vi "GraphAllData.vi"() -> ()   [LabVIEW 2014]
uses:
  <vilib>/Utility/file.llb/Read From Spreadsheet File (DBL).vi
panel:
  in  "Boolean":bool=TRUE caption="Comma - Dot"
  out "Intensity":cluster{dbl[], dbl[]}[](graph)=[{[0.4482, 0.74565, 1.03465, 1.41595, 1.6587500000000002, 2.1205, 2.3416, 2.64395, 2.8270999999999997], [2885.233184799485, 3819.39283016977, 6741.485053135704, 8371.343227868216, 10568.06564807566, 15816.573468461038, 19513.91663154004, 18468.575918850947, 21904.929929348546]}, {[0.7978500000000001, 1.1793, 1.53135, 1.9195, 2.32255, 2.59605, 2.89845, 2.9768, 3.11285], [4913.128828304257, 8837.628945556497, 14162.459131308004, 21909.101985554447, 24670.326730345823, 30736.435346877264, 29659.90767199613, 36470.26711538562, 32082.173989529885]}, {[0.75805, 1.09005, 1.47645, 1.84945, 2.21955, 2.4829000000000003, 2.7510999999999997, 2.9362, 3.0384499999999997], [2427.837864610553, 6520.525680095638, 15723.354958142441, 21679.009604909883, 27664.463875772657, 35328.219444, 30338.40494135966, 36543.11286503484, 32147.938633638245]}, {[0.8815000000000001, 1.2015500000000001, 1.51245, 1.85385, 2.2742999999999998, 2.5146499999999996, 2.71375, 2.854, 2.91995], [6950.989572736701, 14497.805584718632, 20312.386151964263, 34829.46500046118, 46881.37359550876, 60117.265315518525, 64636.230201609826, 64597.35246922127, 64607.68160946114]}]
  in  "Reduce Array Size (2^nTimes)":i32=3
  out "Filenames":string[](array[string])=["ovo-4-Spectrum Jan-07-2022 Time 03-56Analysed #1.and", "ovo-3-Spectrum Jan-07-2022 Time 03-44Analysed #1.and", "ovo-2-Spectrum Jan-07-2022 Time 03-42Analysed #1.and", "ovo-1-Spectrum Jan-07-2022 Time 03-40Analysed #1.and"]
  out "Plot Color":u32[](array[colorbox])=[483491, 16728642, 982784, 4375295]
  in  "Plot.Plot Interpolation":u8=2 max=5
  in  "Plot.Point Style":u8=2 max=16
  in  "Plot.Line Width":u8=5
  in  "Plot.Line Style":u8 max=4
  in  "Length":i32=110
  in  "Start index":i32=33
  out "FWHM":cluster{dbl[], dbl[]}[](graph)=[{[0.4482, 0.74565, 1.03465, 1.41595, 1.6587500000000002, 2.1205, 2.3416, 2.64395, 2.8270999999999997], [34.947243991883, 33.834151010707, 41.858625650798, 28.047486632265, 26.265721513935, 22.606313384127, 20.708480495843, 22.186951698272, 19.059334529408]}, {[0.7978500000000001, 1.1793, 1.53135, 1.9195, 2.32255, 2.59605, 2.89845, 2.9768, 3.11285], [33.067735928078, 24.344505399387, 19.47079873387, 12.074343500554, 15.950722154285, 12.702887849716, 16.078576237118, 9.241305141305, 15.837298026481]}, {[0.75805, 1.09005, 1.47645, 1.84945, 2.21955, 2.4829000000000003, 2.7510999999999997, 2.9362, 3.0384499999999997], [31.856003209472, 17.763577743245, 6.463072800948, 7.100905977113, 6.459600827454, 5.797900738679, 7.140966250209, 6.895364179986, 7.095295071816]}, {[0.8815000000000001, 1.2015500000000001, 1.51245, 1.85385, 2.2742999999999998, 2.5146499999999996, 2.71375, 2.854, 2.91995], [56.013195210149, 21.725458390603, 18.108405137041, 11.925527469703, 8.834451268768, 8.192653465718, 9.670319607355, 12.851225125147, 12.213374983365]}]
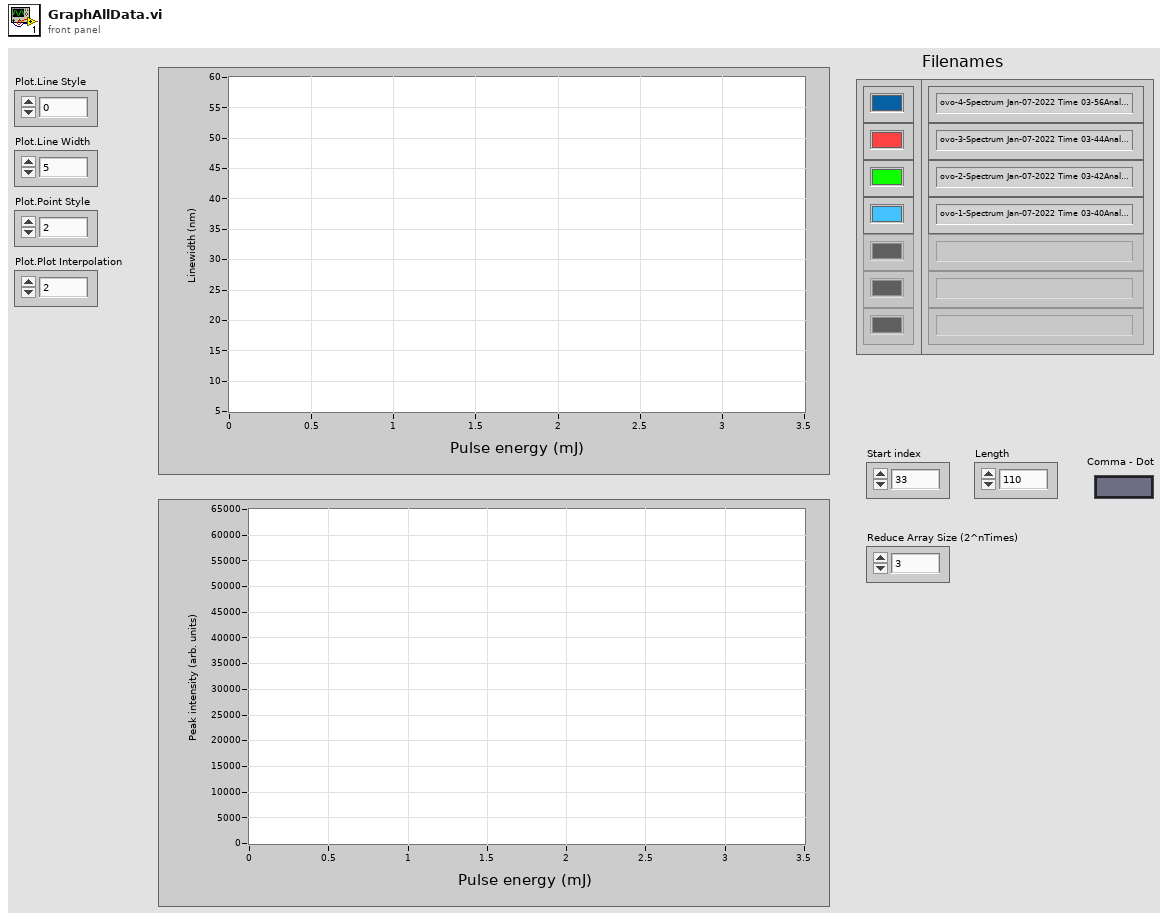
[diagram p1: front panel]
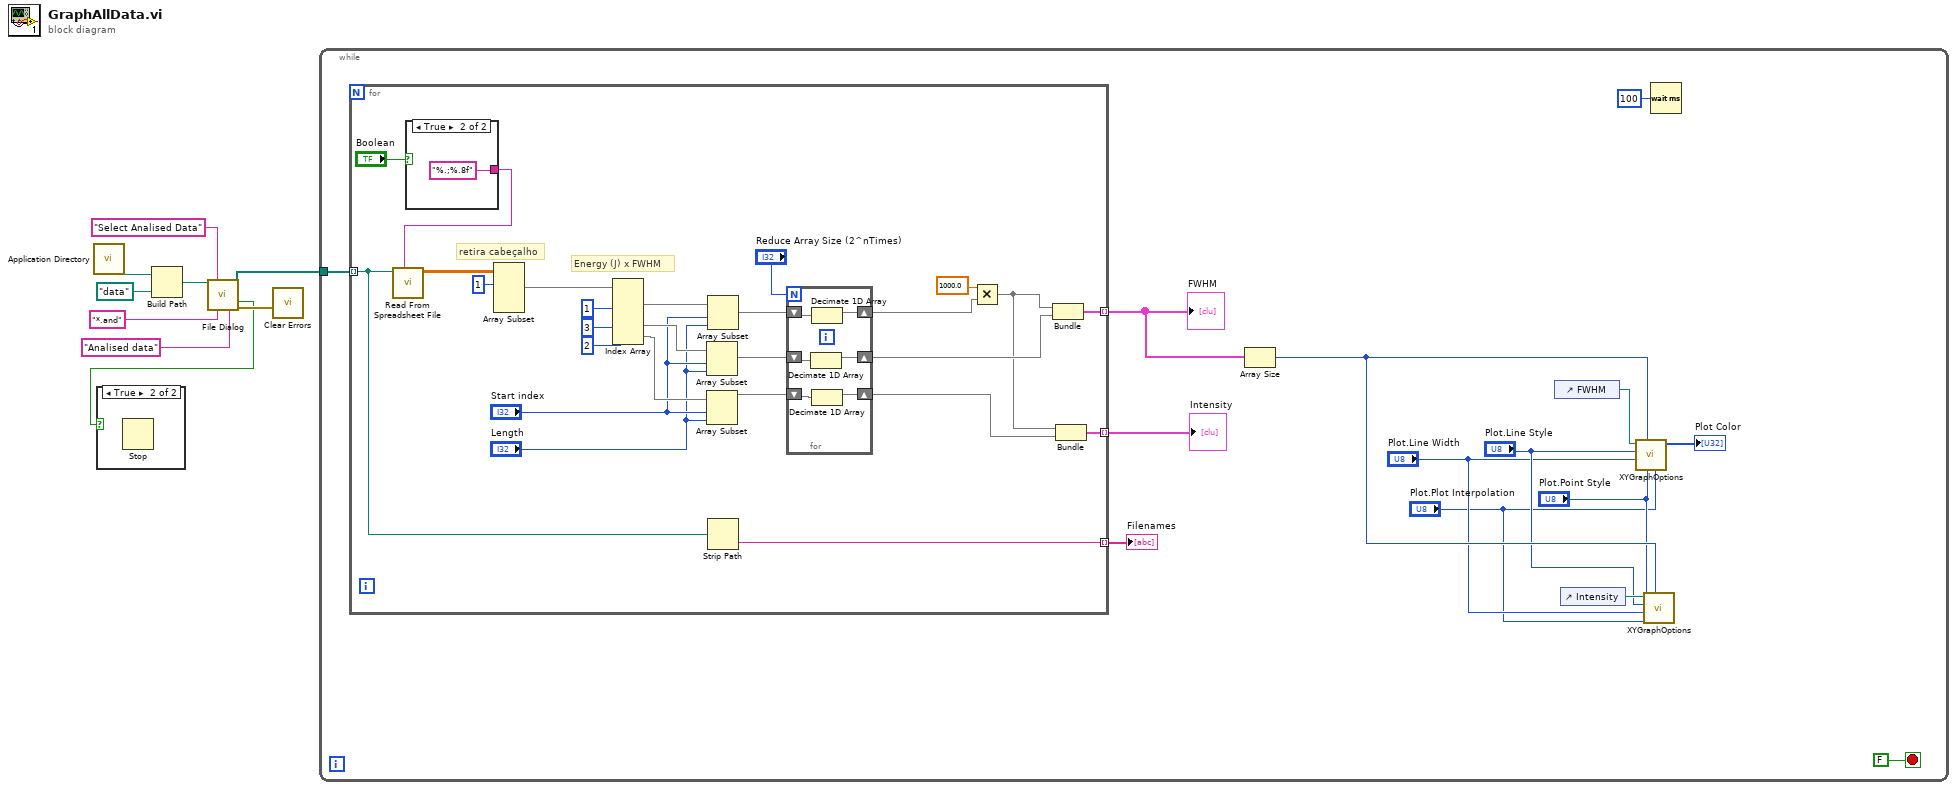
[diagram p0: block diagram]
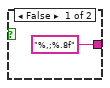
[diagram p2: hidden frame]
diagram:
  n1 = call <vilib>:"Application Directory.vi"() -> ("Application Directory"=w5:path)
  n2 = Build Path(base path=w5, name or relative path=path "data") -> (appended path=w4:path)
  n3 = call "File Dialog"("start path"=w4, "prompt"="Select Analised Data", "pattern (all files)"="*.and", "pattern label"="Analised data") -> ("selected paths"=w1:path[], "cancelled"=w2:bool, "error out"=w3:errorcluster)  [unwired: 8 in, 1 out]
  n4 = case shown="True" w2 {
    frame False {
    }
    frame True {
      n5 = Stop() -> ()  [unwired: 1 in]
    }
  }
  n6 = call <vilib>:"Clear Errors.vi"("error in (no error)"=w3) -> ()  [unwired: 5 in, 2 out]
  n7 = while {
    tunnel: w1 -> [w23]
    stop <- FALSE stop-if-true
    n8 = for {
      tunnel: w23 -> [w40] mode=indexing
      tunnel: [w44] -> w20 mode=indexing
      tunnel: [w39] -> w18 mode=indexing
      tunnel: [w26] -> w16 mode=indexing
      # "Energy (J) x FWHM"
      # "retira cabeçalho"
      n9 = case shown="True" "Boolean" {
        tunnel: ["%,;%.8f" ("format (%.3f)") "%.;%.8f" ("format (%.3f)")] -> w25
        frame False {
        }
        frame True {
        }
      }
      n10 = call-poly <vilib>:"Read From Spreadsheet File.vi"("format (%.3f)"=w25, "file path (dialog if empty)"=w40) -> ("all rows"=w48:dbl[][])  [unwired: 5 in, 4 out]
      n11 = Array Subset(array=w48, index (row)=1 ("index")) -> (w47:dbl[][])  [unwired: 3 in]
      n12 = Index Array(array=w47, index (col) #1=1 ("index (row)"), index (col) #2=3 ("index (col)"), index (col) #3=2 ("index (col)")) -> (element #1=w42:dbl[], element #2=w41:dbl[], element #3=w32:dbl[])  [unwired: 3 in]
      n13 = Array Subset(array=w41, index="Start index", length="Length") -> (w36:dbl[])
      n14 = Array Subset(array=w32, index="Start index", length="Length") -> (w29:dbl[])
      n15 = Array Subset(array=w42, index="Start index", length="Length") -> (w37:dbl[])
      n16 = Strip Path(path=w40) -> (name=w39:string)  [unwired: 1 out]
      n17 = for {
        N: "Reduce Array Size (2^nTimes)" -> [_]
        shift-right: [w55] -> w35
        shift-left: w37 -> [w57]
        shift-right: [w54] -> w34
        shift-left: w36 -> [w56]
        shift-right: [w53] -> w27
        shift-left: w29 -> [w52]
        n18 = Decimate 1D Array(w56) -> (w54:dbl[])  [unwired: 1 out]
        n19 = Decimate 1D Array(w57) -> (w55:dbl[])  [unwired: 1 out]
        n20 = Decimate 1D Array(w52) -> (w53:dbl[])  [unwired: 1 out]
      }
      n21 = Multiply(x=1000.0, y=w35) -> (x*y=w28:dbl[])
      n22 = Bundle(w28, w34) -> (w44:cluster{dbl[], dbl[]})  [unwired: 1 in]
      n23 = Bundle(w28, w27) -> (w26:cluster{dbl[], dbl[]})  [unwired: 1 in]
    }
    "FWHM" <- w20
    "Filenames" <- w18
    "Intensity" <- w16
    n24 = Array Size(array=w20) -> (size(s)=w14:i32)
    n25 = control-ref of="FWHM"() -> (w21:refnum<vi>)
    n26 = control-ref of="Intensity"() -> (w15:refnum<vi>)
    n27 = call "XYGraphOptions.vi"("Plot.Plot Interpolation"="Plot.Plot Interpolation", "Plot.Point Style"="Plot.Point Style", "Numeric Control"=w14, "Plot.Line Width"="Plot.Line Width", "Plot.Line Style"="Plot.Line Style", "XYGraph in"=w21) -> ("Array"=→"Plot Color":u32[])  [unwired: 5 in]
    n28 = call "XYGraphOptions.vi"("Plot.Plot Interpolation"="Plot.Plot Interpolation", "Plot.Point Style"="Plot.Point Style", "Numeric Control"=w14, "Plot.Line Width"="Plot.Line Width", "Plot.Line Style"="Plot.Line Style", "XYGraph in"=w15) -> ()  [unwired: 5 in, 1 out]
    n29 = Wait (ms)(milliseconds to wait=u32 100) -> ()  [unwired: 1 out]
  }
